vi "Write Configuration Parameter.vi"(8 "error in (no error)":errorcluster, 10 "Configuration":T1, 11 "RandomNumberLogger in":refnum<class "RandomNumberLogger.lvclass">) -> (0 "error out":errorcluster, 3 "RandomNumberLogger out":refnum<class "RandomNumberLogger.lvclass">)   [LabVIEW 2020, in "RandomNumberLogger.lvlib" / "RandomNumberLogger.lvclass"]
uses:
  RandomNumberLogger.lvclass
  RandomNumberLogger.lvclass/RandomNumberLogger.ctl
  Configuration.ctl
panel:
  # "#via_ignore"
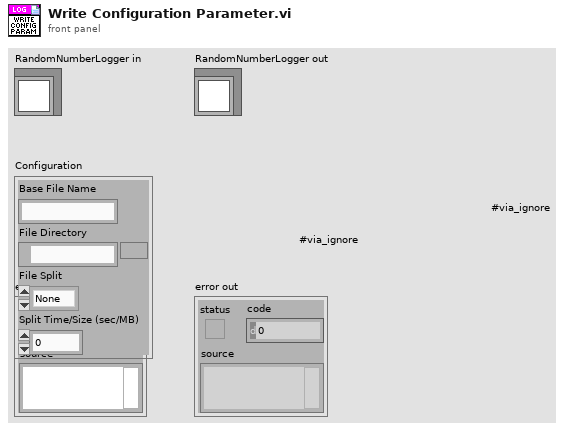
[diagram p1: front panel]
types:
  T1 = typedef "RandomNumberLogger.lvlib/RandomNumberLogger.lvclass/Configuration.ctl" = cluster{"Base File Name":string, "File Directory":path, "File Split":enum16{"None", "Time", "Size"}, "Split Time/Size (sec/MB)":dbl}
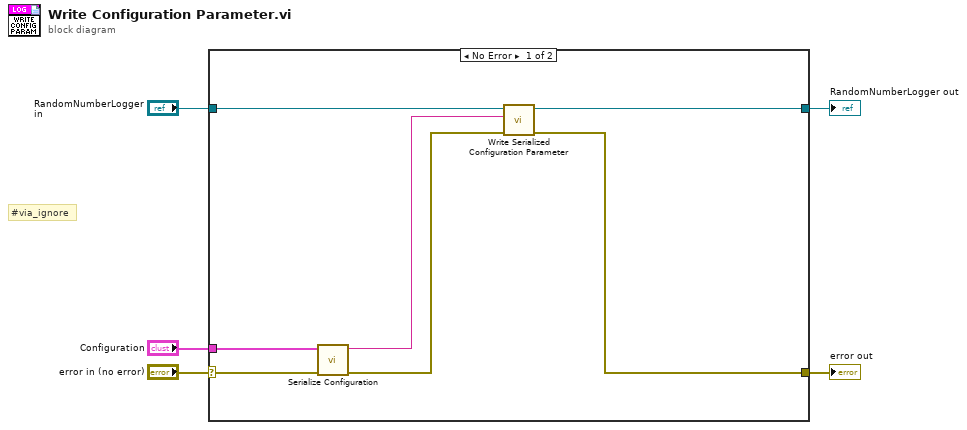
[diagram p0: block diagram]
diagram:
  # "#via_ignore"
  n1 = case shown="No Error" "error in (no error)" {
    selector: "error in (no error)" -> [w10 w14]
    tunnel: [w7 w14] -> w4
    tunnel: [w11 w13] -> w2
    tunnel: "RandomNumberLogger in" -> [w12 w13]
    tunnel: "Configuration" -> [w6 _]
    frame No Error {
      n2 = call "Serialize Configuration.vi"("error in (no error)"=w10, "Configuration"=w6) -> ("error out"=w8:errorcluster, "Serialized Configuration"=w9:string)  [unwired: 8 in]
      n3 = call "Write Serialized Configuration Parameter.vi"("error in (no error)"=w8, "Serialized Configuration"=w9, "RandomNumberLogger in"=w12) -> ("error out"=w7:errorcluster, "RandomNumberLogger out"=w11:refnum<class "RandomNumberLogger.lvclass">)  [unwired: 7 in]
    }
    frame Error {
    }
  }
  "error out" <- w4
  "RandomNumberLogger out" <- w2
